vi "hasProperty.vi"(8 "error in (no error)":errorcluster, 10 "Property Name in":string, 11 "IPropertyObject in":refnum<class "IPropertyObject.lvclass">) -> (0 "error out":errorcluster, 2 "Has Property?":bool, 3 "IPropertyObject out":refnum<class "IPropertyObject.lvclass">)   [LabVIEW 2022 SP3, in "openDAQ.lvlib" / "IBaseObject.lvlib" / "IPropertyObject.lvlib" / "IPropertyObject.lvclass"]
uses:
  <instrlib>/openDAQ/Public/Classes/IPropertyObject/IPropertyObject.lvclass
  <instrlib>/openDAQ/Public/Classes/IPropertyObject/IPropertyObject.lvclass/IPropertyObject.ctl
  <instrlib>/openDAQ/Public/Classes/daqCoreTypes/IString/IString.lvclass
  <instrlib>/openDAQ/Binaries/Windows/x86/copendaq32.dll
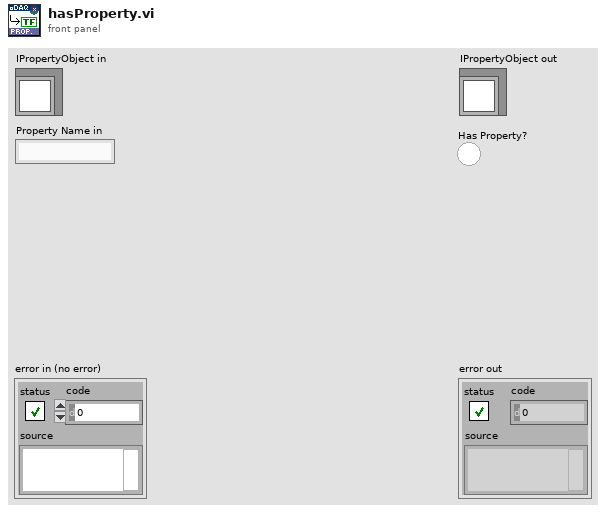
[diagram p1: front panel]
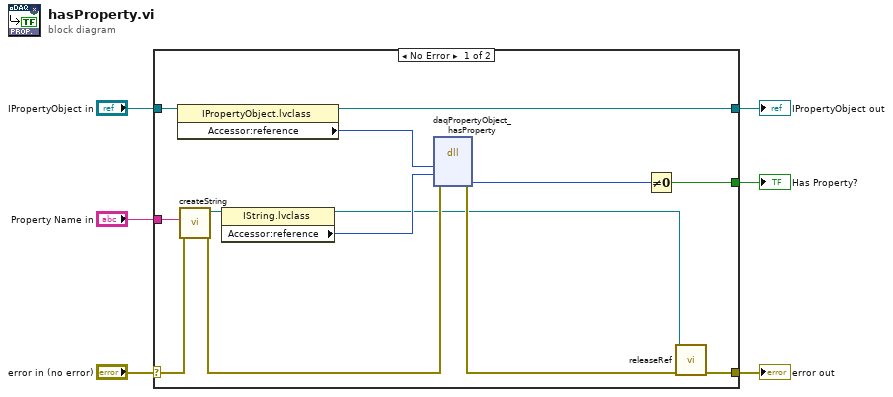
[diagram p0: block diagram]
diagram:
  n1 = case shown="No Error" "error in (no error)" {
    selector: "error in (no error)" -> [w16 w21]
    tunnel: [w11 w21] -> w5
    tunnel: [w17 w20] -> w3
    tunnel: "IPropertyObject in" -> [w19 w20]
    tunnel: "Property Name in" -> [w14 _]
    tunnel: [w7 _] -> w1
    frame No Error {
      n2 = property class="IPropertyObject.lvclass"(reference=w19) -> (reference out=w17:refnum<class "IPropertyObject.lvclass">, "Accessor:reference"=w18:i64)  [unwired: 1 in, 1 out]
      n3 = call <instrlib>:"createString.vi"("error in (no error)"=w16, "String"=w14) -> ("error out"=w15:errorcluster, "IString out"=w13:refnum<class "IString.lvclass">)  [unwired: 8 in]
      n4 = property class="IString.lvclass"(reference=w13) -> (reference out=w9:refnum<class "IString.lvclass">, "Accessor:reference"=w12:i64)  [unwired: 1 in, 1 out]
      n5 = dll-call lib="C:/Program Files (x86)/National Instruments/LabVIEW 2022/instr.lib/openDAQ/Binaries/Windows/x86/copendaq*.*" fn="daqPropertyObject_hasProperty"(error in=w15, "propertyObject"=w18, "name"=w12) -> (error out=w10:errorcluster, "hasProperty"=w8:i32)  [unwired: 6 in, 1 out]
      n6 = Not Equal To 0?(x=w8) -> (x != 0?=w7:bool)
      n7 = call-dynamic "releaseRef.vi"("error in (no error)"=w10, "IBaseObject in"=w9) -> ("error out"=w11:errorcluster)  [unwired: 9 in]
    }
    frame Error {
    }
  }
  "error out" <- w5
  "IPropertyObject out" <- w3
  "Has Property?" <- w1
